vi "Start.vi"(8 "error in (no error)":errorcluster, 11 "MQTT_Base in":refnum<class "MQTT_Base.lvclass">) -> (0 "error out":errorcluster, 1 "timed out?":bool, 3 "MQTT_Base out":refnum<class "MQTT_Base.lvclass">)   [LabVIEW 2013, in "MQTT Base.lvlib" / "MQTT_Base.lvclass"]
uses:
  MQTT_Base.lvclass
  MQTT_Base.lvclass/MQTT_Base.ctl
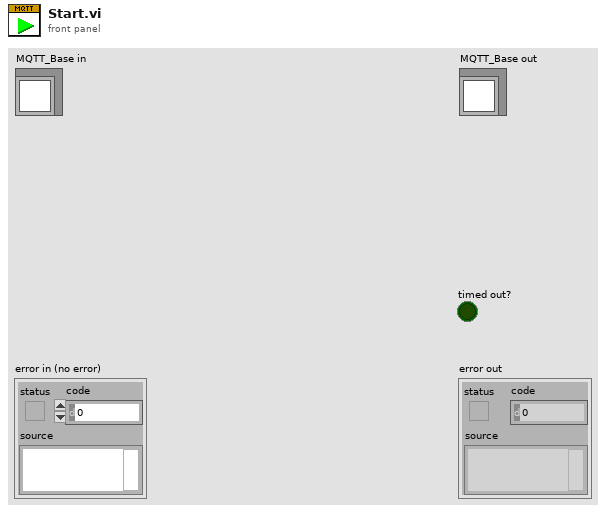
[diagram p1: front panel]
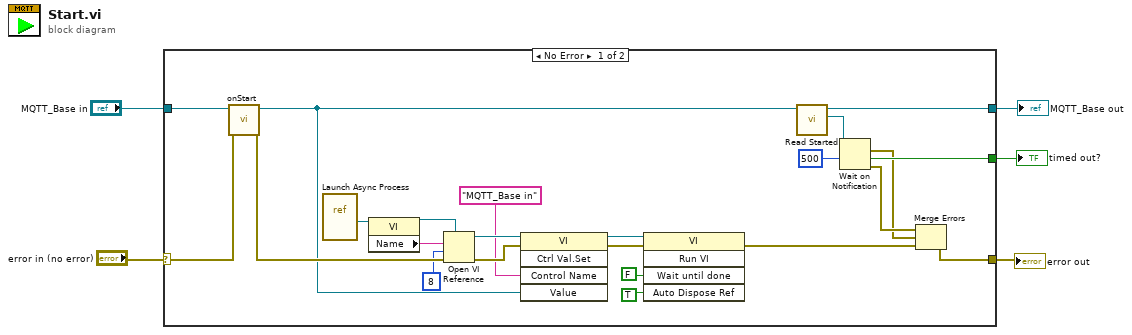
[diagram p0: block diagram]
diagram:
  n1 = case shown="No Error" "error in (no error)" {
    selector: "error in (no error)" -> [w22 w30]
    tunnel: [w24 w30] -> w3
    tunnel: [w19 w29] -> w2
    tunnel: "MQTT_Base in" -> [w23 w29]
    tunnel: [w26 _] -> w1
    frame No Error {
      n2 = call-dynamic "onStart.vi"("error in (no error)"=w22, "MQTT_Base in"=w23) -> ("error out"=w21:errorcluster, "MQTT_Base out"=w17:refnum<class "MQTT_Base.lvclass">)  [unwired: 8 in]
      n3 = vi-ref "Launch Async Process.vi"() -> (w16:refnum<vi>)
      n4 = property class="VI"(reference=w16) -> (reference out=w14:refnum<vi>, "Name"=w15:string)  [unwired: 1 in, 1 out]
      n5 = Open VI Reference(type specifier VI Refnum (for type only)=w14, vi path=w15, options=8, error in (no error)=w21) -> (vi reference=w7:refnum<vi>, error out=w8:errorcluster)  [unwired: 2 in]
      n6 = invoke class="VI" method="Ctrl Val.Set"(reference=w7, error in=w8, "Control Name"="MQTT_Base in", "Value"=w17) -> (reference out=w11:refnum<vi>, error out=w12:errorcluster)  [unwired: 1 in, 3 out]
      n7 = invoke class="VI" method="Run VI"(reference=w11, error in=w12, "Wait until done"=FALSE ("Wait Until Done"), "Auto Dispose Ref"=TRUE ("Auto Dispose Reference")) -> (error out=w18:errorcluster)  [unwired: 1 in, 4 out]
      n8 = call "Read Started.vi"("MQTT_Base in"=w17) -> ("Started"=w25:refnum<notifier>, "MQTT_Base out"=w19:refnum<class "MQTT_Base.lvclass">)  [unwired: 8 in, 1 out]
      n9 = Wait on Notification(notifier=w25, timeout in ms (-1)=500) -> (notification=w20:errorcluster, timed out?=w26:bool, error out=w27:errorcluster)  [unwired: 2 in, 1 out]
      n10 = Merge Errors(w27, w20, w18) -> (w24:errorcluster)
    }
    frame Error {
    }
  }
  "error out" <- w3
  "MQTT_Base out" <- w2
  "timed out?" <- w1
